vi "Untitled 1.vi"() -> ()   [LabVIEW 2017]
panel:
  in  "Boolean 2":bool
  in  "Boolean":bool
  in  "stop":bool
  in  "Path":path
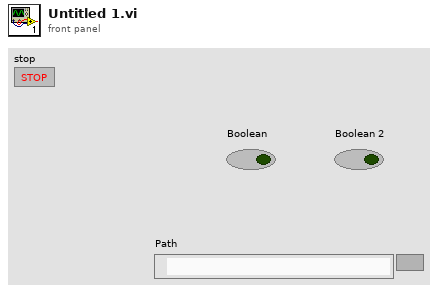
[diagram p1: front panel]
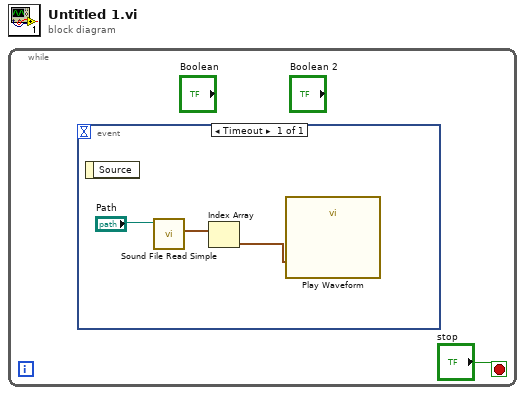
[diagram p0: block diagram]
diagram:
  n1 = while {
    stop <- "stop" stop-if-true
    n2 = event shown="[0] Timeout" {
      selector: _ -> [_]
      dyn-events: _ -> [_]
      timeout: _ -> [_]
      event Timeout {
        n3 = event-data() -> ()  [unwired: 1 in, 1 out]
        n4 = call <vilib>:"Sound File Read Simple.vi"("path"="Path") -> ("data"=w4:waveform(dbl)[])  [unwired: 7 in, 3 out]
        n5 = Index Array(array=w4) -> (element=w3:waveform(dbl))  [unwired: 1 in]
        n6 = call "Play Waveform"("Data"=w3) -> ()  [unwired: 18 in, 1 out]
      }
    }
  }
